vi "Xi^2+Xi-1^2.vi"(10 "X[-1]":dbl, 11 "Xi":dbl[](array[numeric])) -> (3 "Yi":dbl[](array[numeric]) format="%.2f")   [LabVIEW 2012]
doc: "Calculate sums of consecutive array elements. 0th element of output is equal to x(0)+ x(-1), where x(-1) is an optional scalar input that defaults to zero."
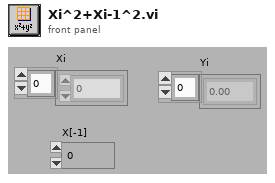
[diagram p1: front panel]
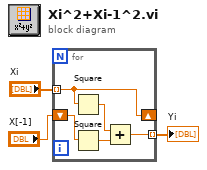
[diagram p0: block diagram]
diagram:
  n1 = for {
    shift-right: [w5] -> _
    shift-left: "X[-1]" -> [w8]
    tunnel: "Xi" -> [w5] mode=indexing
    tunnel: [w4] -> w1 mode=indexing
    n2 = Square(x=w5) -> (x^2=w7:dbl)
    n3 = Square(x=w8) -> (x^2=w6:dbl)
    n4 = Add(x=w7, y=w6) -> (x+y=w4:dbl)
  }
  "Yi" <- w1
